vi "Correlation.vi"() -> ()   [LabVIEW 2014]
uses:
  <vilib>/Platform/TimedLoop/XDataNode/timing_clust.ctl
  <vilib>/Platform/TimedLoop/XDataNode/nitl_modes.ctl
  <vilib>/Platform/TimedLoop/XDataNode/wakeup.ctl
  <vilib>/myRIO/Instrument Drivers/Onboard IO/AI/typedefs/AI Reference.ctl
  <vilib>/myRIO/Common/Instrument Driver Framework/Utilities/typedefs/myRIO Generic Hardware Reference.ctl
  <vilib>/myRIO/Common/Instrument Driver Framework/Utilities/typedefs/Hardware Version Enum.ctl
  <vilib>/myRIO/Common/Instrument Driver Framework/Utilities/typedefs/myRIO v1.0 Reference.ctl
  <vilib>/myRIO/Common/Instrument Driver Framework/Utilities/typedefs/Generic FPGA Reference.ctl
  <vilib>/myRIO/Common/Instrument Driver Framework/myRIO v1.0/AI/typedefs/AI Channels List.ctl
  <vilib>/myRIO/Common/Instrument Driver Framework/myRIO v1.0/AI/typedefs/AI Channels Enum.ctl
  <vilib>/myRIO/Common/Instrument Driver Framework/Utilities/typedefs/Analog Scaling Constants List.ctl
  <vilib>/myRIO/Common/Instrument Driver Framework/Utilities/typedefs/Analog Scaling Constants.ctl
  <vilib>/userdefined/High Color/nirio_resource_hc.ctl
  <vilib>/myRIO/Instrument Drivers/Onboard IO/DIO/typedefs/DIO Reference.ctl
  <vilib>/myRIO/Common/Instrument Driver Framework/myRIO v1.0/DIO/typedefs/DIO Channels List.ctl
  <vilib>/myRIO/Common/Instrument Driver Framework/myRIO v1.0/DIO/typedefs/DIO Channels Enum.ctl
  <vilib>/myRIO/Common/Instrument Driver Framework/Utilities/vis/Is FPGA Ref Available.vi
  <vilib>/myRIO/Common/Instrument Driver Framework/myRIO v1.0/AI/vis/myRIO v1.1 Open AI.vi
  <vilib>/myRIO/Instrument Drivers/Onboard IO/AI/vis/Read.vi
  <vilib>/myRIO/Common/Instrument Driver Framework/myRIO v1.0/DIO/vis/myRIO v1.1 Open DIO.vi
  <vilib>/myRIO/Instrument Drivers/Onboard IO/DIO/vis/Write.vi
  <vilib>/myRIO/Common/Instrument Driver Framework/Utilities/vis/Validate Channels.vi
  <vilib>/myRIO/Common/Instrument Driver Framework/myRIO v1.0/AI/vis/myRIO v1.0 Reserve AI.vi
  <vilib>/myRIO/Common/Instrument Driver Framework/myRIO v1.0/DIO/vis/myRIO v1.0 Reserve DIO.vi
  <vilib>/myRIO/Common/Instrument Driver Framework/myRIO v1.0/AI/vis/myRIO v1.0 Build MUX Configuration AI.vi
  <vilib>/myRIO/Common/Instrument Driver Framework/myRIO v1.0/Resource Manager/vis/myRIO v1.0 Reserve Channel List.vi
  <vilib>/myRIO/Common/Instrument Driver Framework/myRIO v1.0/DIO/vis/myRIO v1.0 Build MUX Configuration DIO.vi
  <vilib>/myRIO/Common/Instrument Driver Framework/myRIO v1.0/Resource Manager/vis/myRIO v1.0 Reserve Channel.vi
  <vilib>/myRIO/Common/Instrument Driver Framework/myRIO v1.0/Resource Manager/vis/myRIO v1.0 Unreserve Channel.vi
  <vilib>/myRIO/Common/Instrument Driver Framework/myRIO v1.0/Resource Manager/vis/myRIO v1.0 Create Configuration List.vi
  <vilib>/myRIO/Common/Instrument Driver Framework/myRIO v1.0/Resource Manager/vis/myRIO v1.0 Build Mutex Name.vi
  <vilib>/Utility/VariantDataType/GetNumericInfo.vi
  <vilib>/Utility/error.llb/Error Cluster From Error Code.vi
  <vilib>/myRIO/Common/Instrument Driver Framework/myRIO v1.0/myRIO v1.1 Open.vi
  <vilib>/myRIO/Common/Instrument Driver Framework/myRIO v1.0/AI/vis/myRIO v1.0 Get Scaling Constants AI.vi
  <vilib>/myRIO/Common/Instrument Driver Framework/Utilities/vis/IO Manager.vi
  <vilib>/myRIO/Common/Instrument Driver Framework/Utilities/vis/Configuration Manager.vi
  <vilib>/myRIO/Common/Instrument Driver Framework/myRIO v1.0/myRIO v1.0 Close.vi
  <vilib>/myRIO/Common/Instrument Driver Framework/myRIO v1.0/AI/vis/myRIO v1.0 Read AI.vi
  <vilib>/myRIO/Common/Instrument Driver Framework/myRIO v1.0/Resource Manager/vis/myRIO v1.0 Configure IO.vi
  <vilib>/myRIO/Common/Instrument Driver Framework/myRIO v1.0/DIO/vis/myRIO v1.0 Write DIO.vi
  <vilib>/platform/TimedLoop/XDataNode/XDataNode.xnode
  <vilib>/myRIO/Express VI/Onboard IO/AI/AI Express VI.xnode
  <vilib>/myRIO/Instrument Drivers/Onboard IO/AI/vis/myRIO AI Open.xnode
  <vilib>/myRIO/Express VI/Onboard Devices/LED/LED Express VI.xnode
  <vilib>/myRIO/Instrument Drivers/Onboard IO/DIO/vis/myRIO DIO Open.xnode
  <vilib>/Platform/TimedLoop/XDataNode/XDNodeRunTimeDep.lvlib
  <vilib>/myRIO/Instrument Drivers/Onboard IO/AI/AI.lvlib
  <vilib>/myRIO/Instrument Drivers/Onboard IO/DIO/DIO.lvlib
panel:
  in  "Window Length":i32=200
  out "error out":errorcluster
  in  "Stop Button":bool
  out "Input signal":dbl[](graph)=[-0.003662109, -0.001220703, -0.001220703, -0.003662109, -0.002441406, -0.002441406, -0.003662109, -0.003662109, -0.003662109, -0.003662109, -0.002441406, -0.003662109, -0.003662109, -0.002441406, -0.003662109, -0.006103515, -0.004882812, -0.003662109, -0.003662109, -0.003662109, -0.002441406, -0.006103515, -0.003662109, -0.001220703, -0.001220703, -0.002441406, -0.002441406, -0.003662109, -0.004882812, -0.003662109, -0.003662109, -0.003662109, -0.003662109, -0.003662109, -0.004882812, -0.006103515, -0.003662109, -0.003662109, -0.002441406, -0.002441406, -0.002441406, -0.006103515, -0.002441406, -0.003662109, -0.003662109, -0.002441406, -0.007324218, -0.003662109, -0.003662109, -0.003662109, -0.004882812, -0.003662109, -0.003662109, -0.003662109, -0.003662109, -0.003662109, -0.002441406, -0.002441406, -0.003662109, -0.003662109, -0.003662109, -0.003662109, -0.006103515, -0.003662109, -0.002441406, -0.002441406, -0.004882812, -0.004882812, -0.003662109, -0.001220703, -0.004882812, -0.003662109, -0.002441406, -0.002441406, -0.004882812, -0.003662109, -0.002441406, -0.003662109, -0.004882812, -0.003662109, -0.003662109, -0.002441406, -0.003662109, -0.003662109, -0.001220703, -0.002441406, -0.004882812, -0.003662109, -0.004882812, -0.003662109, -0.003662109, -0.002441406, -0.002441406, -0.006103515, -0.003662109, -0.003662109, -0.002441406, -0.002441406, -0.002441406, -0.006103515, -0.004882812, -0.003662109, -0.002441406, -0.006103515, -0.006103515, 0.0, -0.003662109, -0.003662109, -0.004882812, -0.006103515, -0.003662109, -0.002441406, -0.002441406, -0.003662109, -0.006103515, -0.006103515, -0.004882812, -0.004882812, -0.002441406, -0.002441406, -0.002441406, -0.003662109, -0.006103515, -0.003662109, -0.002441406, -0.003662109, -0.003662109, -0.002441406, -0.003662109, -0.003662109, -0.004882812, -0.003662109, -0.003662109, -0.004882812, -0.004882812, -0.003662109, -0.002441406, -0.003662109, -0.003662109, -0.003662109, -0.003662109, -0.004882812, -0.006103515, -0.003662109, -0.002441406, -0.003662109, -0.004882812, -0.003662109, -0.003662109, -0.003662109, -0.003662109, -0.002441406, -0.002441406, -0.003662109, -0.003662109, -0.003662109, -0.002441406, -0.002441406, -0.006103515, -0.003662109, -0.002441406, -0.002441406, -0.003662109, -0.002441406, -0.002441406, -0.003662109, -0.003662109, -0.003662109, -0.003662109, -0.003662109, -0.002441406, -0.006103515, -0.006103515, -0.003662109, -0.002441406, -0.006103515, -0.006103515, -0.002441406, -0.002441406, -0.002441406, -0.004882812, -0.003662109, -0.002441406, -0.002441406, -0.004882812, -0.002441406, -0.003662109, -0.003662109, -0.003662109, -0.003662109, -0.002441406, -0.004882812, -0.003662109, -0.003662109, -0.002441406, -0.003662109, -0.003662109, -0.004882812, -0.002441406, -0.001220703, -0.003662109]
  in  "Period \n(microseconds)":i64=1000
  in  "Frequency4":dbl=941.0
  in  "Frequency3":dbl=852.0
  in  "Frequency2":dbl=770.0
  in  "Frequency1":dbl=697.0
  in  "Threshold":dbl
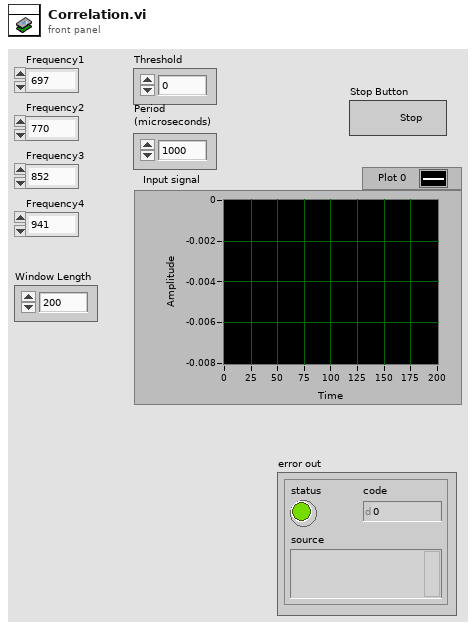
[diagram p1: front panel]
types:
  T1 = typedef "DIO.lvlib/DIO Reference.ctl" = cluster{"myRIO Reference":T2, "DIO Channels List":T6}
  T2 = typedef "myRIO Generic Hardware Reference.ctl" = cluster{"myRIO Model":T3, "myRIO Hardware Reference":T4}
  T3 = typedef "Hardware Version Enum.ctl" = enum16{"Unknown", "myRIO-1900", "myRIO-1950"}
  T4 = typedef "myRIO v1.0 Reference.ctl" = cluster{"Generic FPGA Reference":T5, "Allow multiple opens":bool}
  T5 = typedef "Generic FPGA Reference.ctl" = refnum<k20>
  T6 = typedef "DIO Channels List.ctl" = T7[]
  T7 = typedef "DIO Channels Enum.ctl" = enum16{"Not Connected", "C/DIO0", "C/DIO1", "C/DIO2", "C/DIO3", "C/DIO4", "C/DIO5", "C/DIO6", "C/DIO7", "A/DIO0", "A/DIO1", "A/DIO2", "A/DIO3", "A/DIO4", "A/DIO5", "A/DIO6", "A/DIO7", "A/DIO8", "A/DIO9", "A/DIO10", "A/DIO11", "A/DIO12", "A/DIO13", "A/DIO14", "A/DIO15", "B/DIO0", "B/DIO1", "B/DIO2", "B/DIO3", "B/DIO4", "B/DIO5", "B/DIO6", "B/DIO7", "B/DIO8", "B/DIO9", "B/DIO10", "B/DIO11", "B/DIO12", "B/DIO13", "B/DIO14", "B/DIO15", "LED0", "LED1", "LED2", "LED3", "Button0"}
  T8 = typedef "nirio_resource_hc.ctl" = tag
  T9 = typedef "AI.lvlib/AI Reference.ctl" = cluster{"myRIO Reference":T2, "AI Channels List":T10, "AI Scaling Constants List":T12}
  T10 = typedef "AI Channels List.ctl" = T11[]
  T11 = typedef "AI Channels Enum.ctl" = enum16{"Not Connected", "AudioIn/Left", "AudioIn/Right", "C/AI0", "C/AI1", "A/AI0", "A/AI1", "A/AI2", "A/AI3", "B/AI0", "B/AI1", "B/AI2", "B/AI3"}
  T12 = typedef "Analog Scaling Constants List.ctl" = T13[]
  T13 = typedef "Analog Scaling Constants.ctl" = cluster{"LSB Weight (Volts)":dbl, "Offset (Volts)":dbl, "Signed?":bool}
  T14 = typedef "XDNodeRunTimeDep.lvlib/timing_clust.ctl" = cluster{"Expected End [f-1]":u64, "Actual End [f-1]":u64, "Finished Late? [f-1]":bool, "Expected End [i-1]":u64, "Actual End [i-1]":u64, "Finished Late? [i-1]":bool, "Expected Start [i]":u64, "Actual Start [i]":u64, "Expected Start [f]":u64, "Actual Start [f]":u64, "Source Name":string, "Structure Name":string, "Period":i64, "Deadline":i64, "Offset":i64, "Start":i64, "Priority":i32, "Timeout":i32, "Mode":T15, "Wakeup Reason":T16, "Error":errorcluster, "Source Type":string, "Secondary Source Type":string, "Global End Time":u64, "Global Start Time":u64, "Frame Duration":u64, "Iteration Duration":u64, "Assigned CPU":i32, "I/O Scan Engine Mode":u32}
  T15 = typedef "XDNodeRunTimeDep.lvlib/nitl_modes.ctl" = enum32{"No Change", "Process missed periods, maintain original phase", "Discard missed periods, maintain original phase", "Process missed periods, ignore original phase", "Discard missed periods, ignore original phase"}
  T16 = typedef "XDNodeRunTimeDep.lvlib/wakeup.ctl" = enum32{"Normal", "Aborted", "Asynchronous wakeup", "Timing source error", "Timed loop error", "Timeout"}
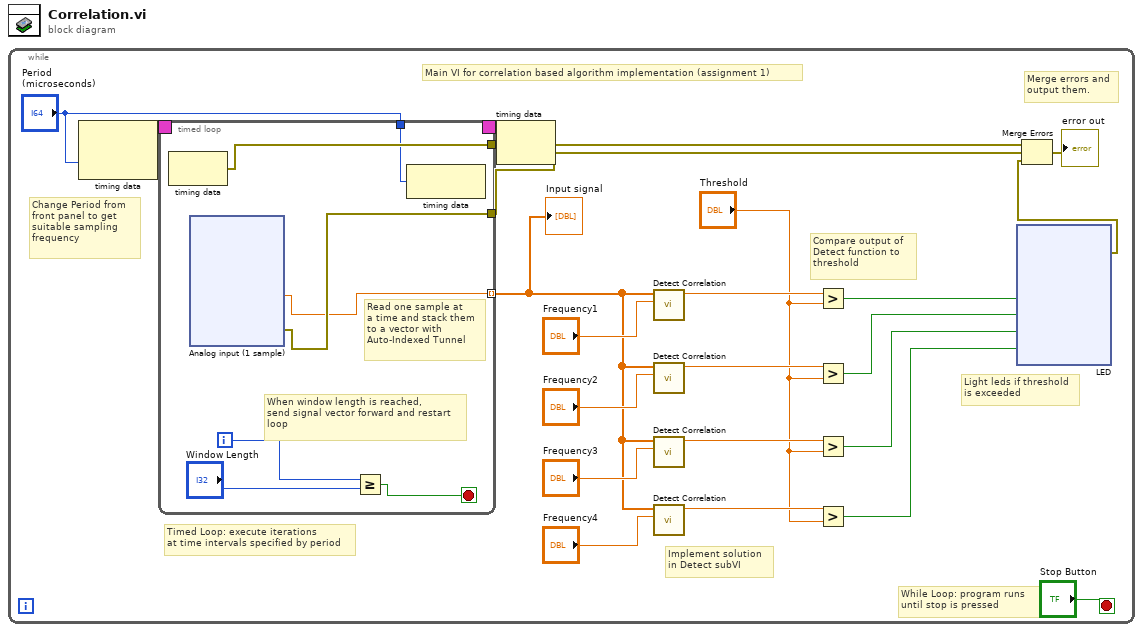
[diagram p0: block diagram]
diagram:
  n1 = while {
    stop <- "Stop Button" stop-if-true
    # "Main VI for correlation based algorithm implementation (assignment 1)"
    # "Light leds if threshold\nis exceeded"
    # "Change Period from\nfront panel to get\nsuitable sampling \nfrequency"
    # "Implement solution\nin Detect subVI"
    # "Timed Loop: execute iterations\nat time intervals specified by period"
    # "Compare output of\nDetect function to \nthreshold"
    # "Merge errors and\noutput them."
    # "While Loop: program runs\nuntil stop is pressed"
    n2 = node-c288("Period \n(microseconds)") -> (w22:T14)  [unwired: 1 in]
    n3 = timed-loop {
      timing: w22 -> [_]
      timing-out: [_] -> w21
      tunnel: [w62] -> w11 mode=indexing
      tunnel: [w67] -> _
      tunnel: [w63] -> w7
      tunnel: "Period \n(microseconds)" -> [w61]
      i -> [w66]
      stop <- w64 stop-if-true
      # "When window length is reached,\nsend signal vector forward and restart\nloop"
      # "Read one sample at \na time and stack them\nto a vector with \nAuto-Indexed Tunnel"
      n4 = node-c288() -> (w67:errorcluster)  [unwired: 1 in]
      n5 = xnode "Analog input (1 sample)"() -> ("AudioIn/Left"=w62:dbl, "error out"=w63:errorcluster)  [unwired: 1 in]
      n6 = Greater Or Equal?(x=w66, y="Window Length") -> (x >= y?=w64:bool)
      n7 = node-c288(w61) -> ()  [unwired: 1 out]
    }
    "Input signal" <- w11
    n8 = node-c288(w21) -> (w8:errorcluster)
    n9 = call "Detect Correlation.vi"("frequency"="Frequency1", "Signal"=w11) -> ("Output"=w20:dbl)  [unwired: 9 in]
    n10 = call "Detect Correlation.vi"("frequency"="Frequency2", "Signal"=w11) -> ("Output"=w15:dbl)  [unwired: 9 in]
    n11 = call "Detect Correlation.vi"("frequency"="Frequency3", "Signal"=w11) -> ("Output"=w14:dbl)  [unwired: 9 in]
    n12 = call "Detect Correlation.vi"("frequency"="Frequency4", "Signal"=w11) -> ("Output"=w13:dbl)  [unwired: 9 in]
    n13 = Greater?(x=w20, y="Threshold") -> (0:w5:bool)
    n14 = Greater?(x=w15, y="Threshold") -> (0:w4:bool)
    n15 = Greater?(x=w14, y="Threshold") -> (0:w3:bool)
    n16 = Greater?(x=w13, y="Threshold") -> (0:w2:bool)
    n17 = xnode "LED"("LED0"=w5, "LED1"=w4, "LED2"=w3, "LED3"=w2) -> ("error out"=w6:errorcluster)  [unwired: 1 in]
    n18 = Merge Errors(w8, w7, w6) -> (→"error out":errorcluster)
  }
